vi "Simulate iRobot Drive.vi"(8 "error in":errorcluster, 9 "Left Wheel Speed (mm/s)":dbl(slide) scale=-500.0..500.0, 10 "Right Wheel Speed (mm/s)":dbl(slide) scale=-500.0..500.0, 11 "Cal Climber":T1) -> (0 "error out":errorcluster, 3 "Cal Climber":T1)   [LabVIEW 2013]
uses:
  Simulate iRobot.ctl
  <instrlib>/DC Motor Controller/HAIOL/DC Motor Controller.lvclass
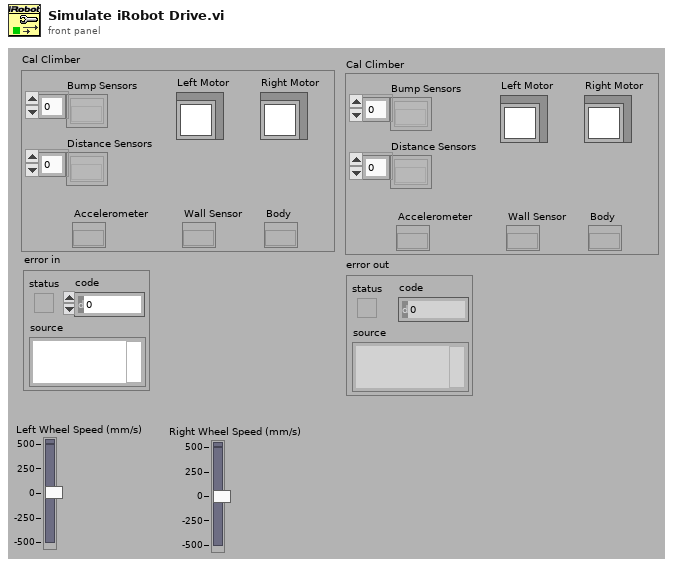
[diagram p1: front panel]
types:
  T1 = typedef "Simulate iRobot.ctl" = cluster{"Bump Sensors":refnum<k20>[], "Distance Sensors":refnum<k20>[], "Accelerometer":refnum<k20>, "Wall Sensor":refnum<k20>, "Body":refnum<k20>, "Left Motor":refnum<class "DC Motor Controller.lvclass">, "Right Motor":refnum<class "DC Motor Controller.lvclass">}
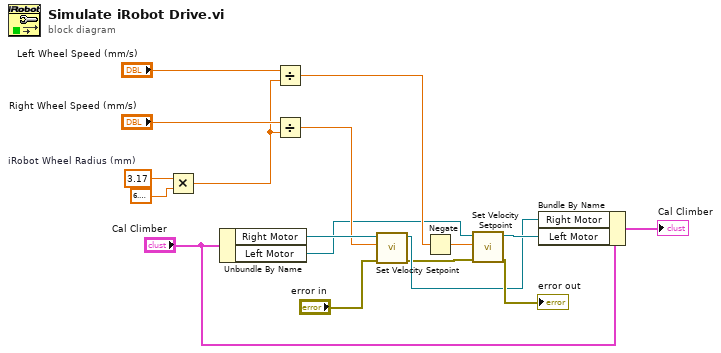
[diagram p0: block diagram]
diagram:
  w12 = 3.17  # iRobot Wheel Radius (mm)
  n1 = Multiply(x=w12, y=6.283185307179586) -> (x*y=w10:dbl)
  n2 = Unbundle By Name("Cal Climber") -> ("Right Motor"=w9:refnum<class "DC Motor Controller.lvclass">, "Left Motor"=w6:refnum<class "DC Motor Controller.lvclass">)
  n3 = Divide(x="Left Wheel Speed (mm/s)", y=w10) -> (x/y=w16:dbl)
  n4 = Divide(x="Right Wheel Speed (mm/s)", y=w10) -> (x/y=w8:dbl)
  n5 = call-dynamic "Set Velocity Setpoint.vi"("error in (no error)"="error in", "CCW Velocity (0 rad/s)"=w8, "DC Motor Controller in"=w9) -> ("error out"=w1:errorcluster, "DC Motor Controller out"=w2:refnum<class "DC Motor Controller.lvclass">)  [unwired: 7 in]
  n6 = Negate(x=w16) -> (-x=w5:dbl)
  n7 = call-dynamic "Set Velocity Setpoint.vi"("error in (no error)"=w1, "CCW Velocity (0 rad/s)"=w5, "DC Motor Controller in"=w6) -> ("error out"=→"error out":errorcluster, "DC Motor Controller out"=w3:refnum<class "DC Motor Controller.lvclass">)  [unwired: 7 in]
  n8 = Bundle By Name(cluster="Cal Climber", "Right Motor"=w2, "Left Motor"=w3) -> (→"Cal Climber":T1)
